vi "auto auger.vi"(3 "Number of Frisbees":i8, 4 "Index Down":bool, 5 "Index Up":bool) -> (0 "Number of Frisbees Out":i8, 1 "Setpoint Out":dbl format="%.2f", 2 "Finished":bool)   [LabVIEW 2012]
uses:
  typedefs/subStates.ctl
  <vilib>/addons/control/pid/NI_PID_pid.lvlib
  <vilib>/addons/control/pid/pid.llb/PID (DBL).vi
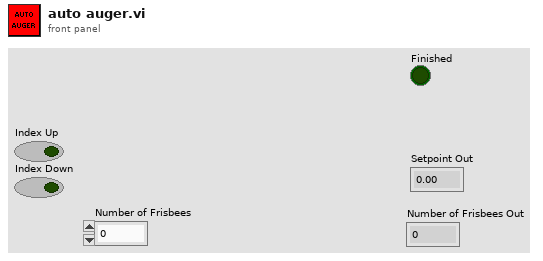
[diagram p1: front panel]
types:
  T1 = typedef "subStates.ctl" = enum16{"null", "wait", "driver control", "auto", "manual override", "hold position", "rotate", "feeder", "shoot", "end"}
  T2 = typedef "WPI_DigitalInputDevRef.ctl" = cluster{"DevStatus":errorcluster, "DIO Channel":T3, "Digital Module":T4}
  T3 = typedef "FPGA_DIOChannel.ctl" = enum8{"DIO 1", "DIO 2", "DIO 3", "DIO 4", "DIO 5", "DIO 6", "DIO 7", "DIO 8", "DIO 9", "DIO 10", "DIO 11", "DIO 12", "DIO 13", "DIO 14", "Invalid"}
  T4 = typedef "FPGA_TypedefDigitalModule.ctl" = enum16{"Digital Module 1", "Digital Module 2"}
  T5 = typedef "WPI_EncoderDevRef.ctl" = cluster{"DevStatus":errorcluster, "EncoderIndex":T6, "CounterIndex":T7, "DistancePerCount":dbl, "Decoding Type":T8}
  T6 = typedef "FPGA_EncoderIdx.ctl" = enum8{"Enc 0", "Enc 1", "Enc 2", "Enc 3", "Invalid"}
  T7 = typedef "FPGA_CounterCtrSystemIndex.ctl" = enum8{"Ctr 0", "Ctr 1", "Ctr 2", "Ctr 3", "Ctr 4", "Ctr 5", "Ctr 6", "Ctr 7", "Invalid"}
  T8 = typedef "WPI_EncoderType.ctl" = enum16{"1x", "2x", "4x"}
  T9 = cluster{"proportional gain (Kc)":dbl, "integral time (Ti, min)":dbl, "derivative time (Td, min)":dbl}
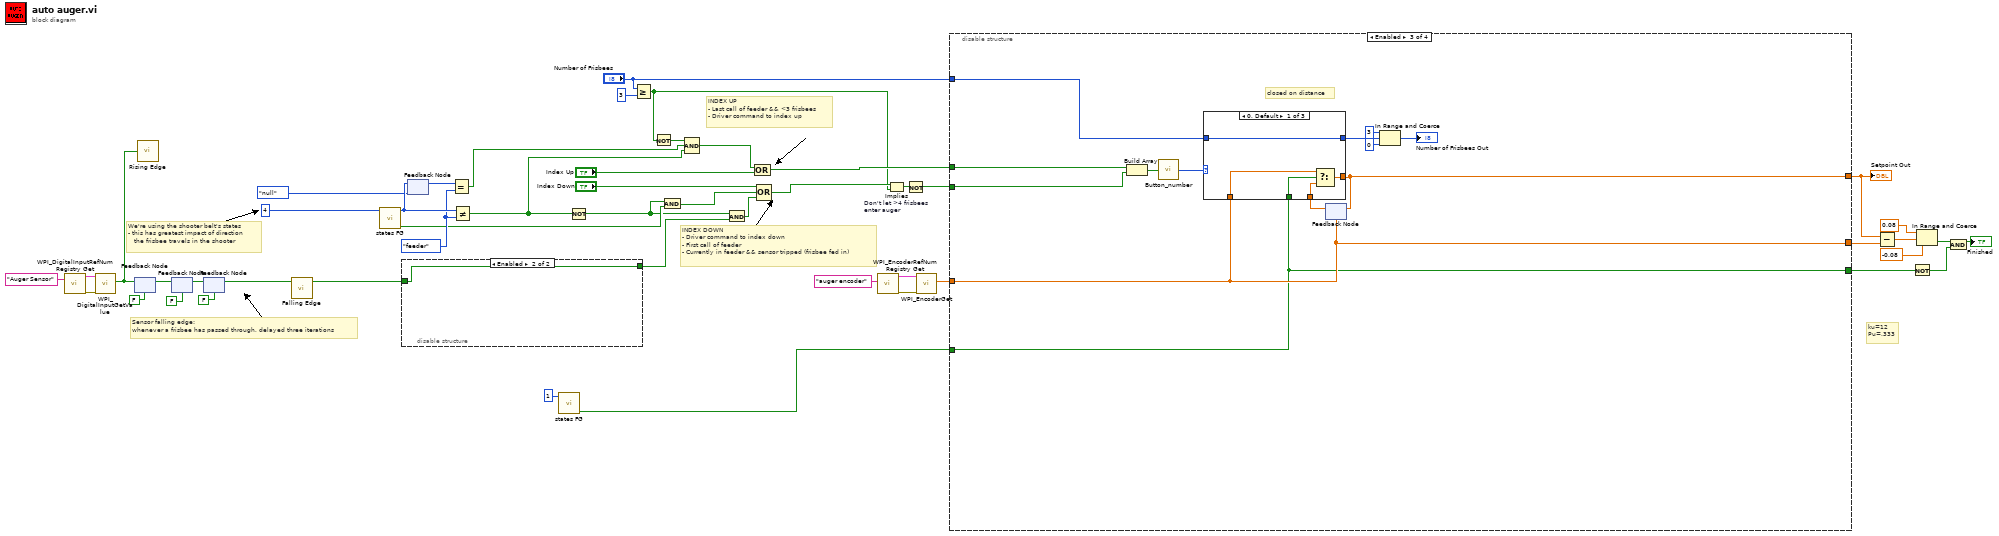
[diagram p0: block diagram]
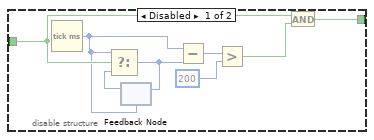
[diagram p2: hidden frame]
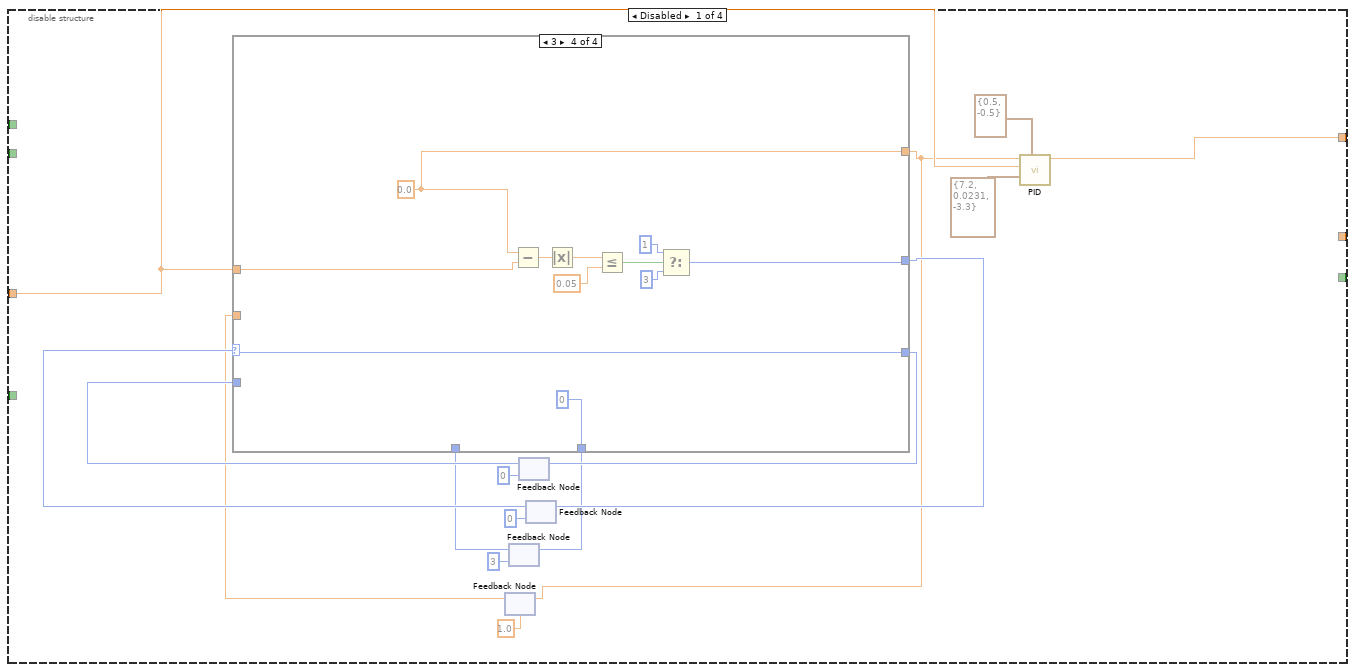
[diagram p3: hidden frame]
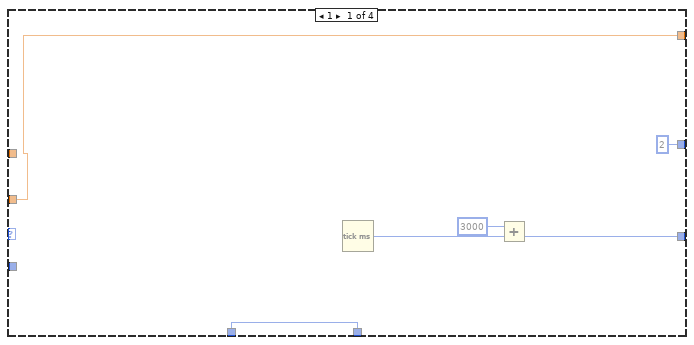
[diagram p4: hidden frame]
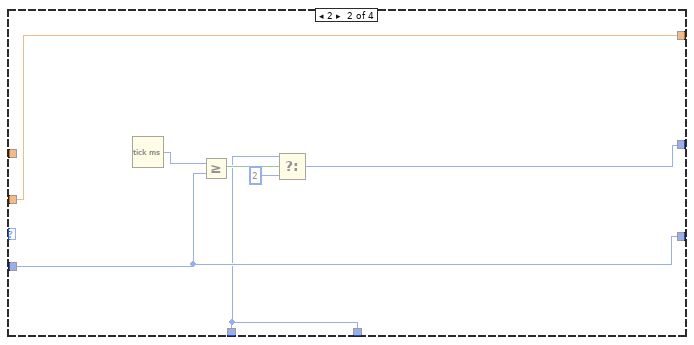
[diagram p5: hidden frame]
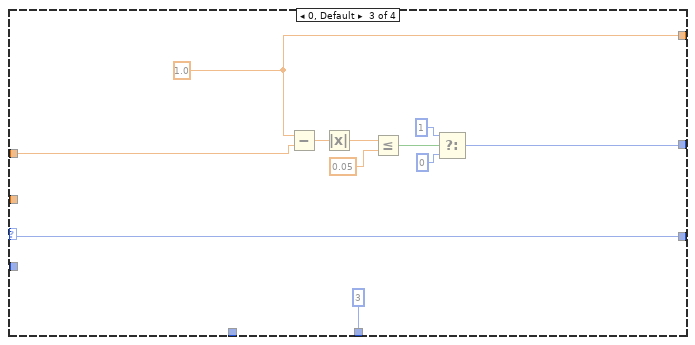
[diagram p6: hidden frame]
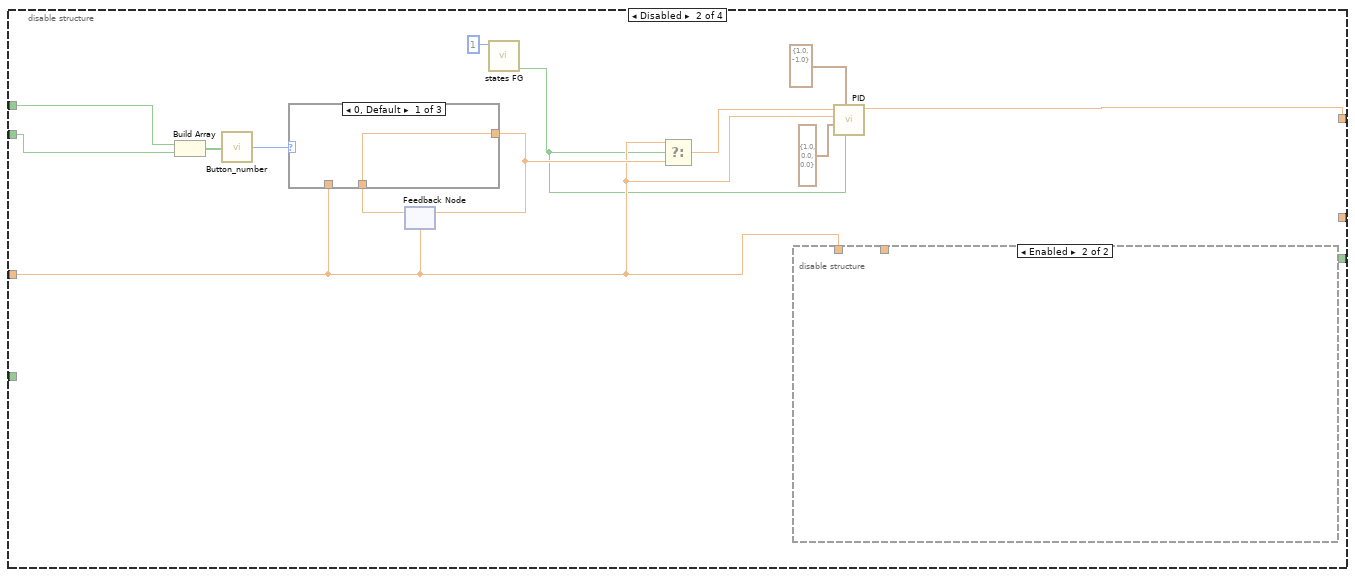
[diagram p7: hidden frame]
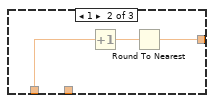
[diagram p8: hidden frame]
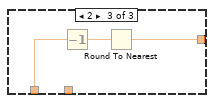
[diagram p9: hidden frame]
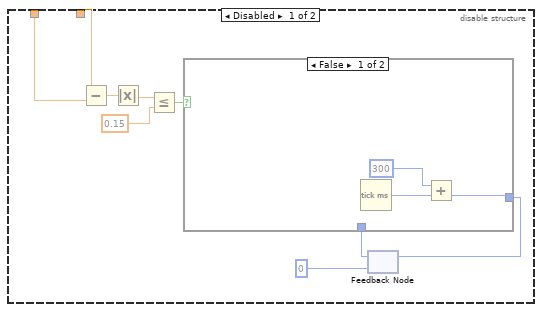
[diagram p10: hidden frame]
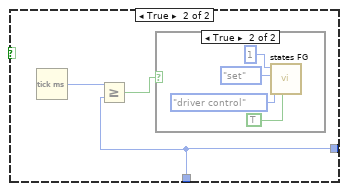
[diagram p11: hidden frame]
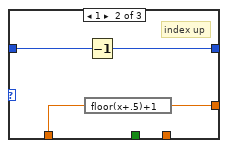
[diagram p13: hidden frame]
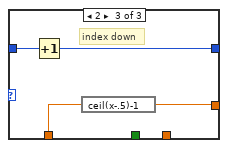
[diagram p14: hidden frame]
diagram:
  w36 = subStates."feeder" ("x")
  # "Sensor falling edge:\nwhenever a frisbee has passed through, delayed three iterations"
  # "We're using the shooter belt's states\n- this has greatest impact of direction\n   the frisbee travels in the shooter"
  # "INDEX DOWN\n- Driver command to index down\n- First call of feeder\n- Currently in feeder && sensor tripped (frisbee fed in)"
  # "INDEX UP\n- Last call of feeder && <3 frisbees\n- Driver command to index up"
  # "ku=12\nPu=.333"
  n1 = call <vilib>:"WPI_DigitalInputRefNum Registry Get.vi"("refnum name"="Auger Sensor") -> ("error out"=w42:errorcluster, "DigitalInputDevRef"=w41:T2)  [unwired: 9 in]
  n2 = call <vilib>:"WPI_DigitalInputGetValue.vi"("error in (no error)"=w42, "DigitalInputDevRef"=w41) -> ("Value"=w15:bool)  [unwired: 7 in, 2 out]
  n3 = feedback-in #1(w15) -> ()
  n4 = feedback #1(FALSE) -> (w19:bool)
  n5 = call "Rising Edge.vi"("Input"=w15) -> ()  [unwired: 1 out]
  n6 = feedback #2(FALSE) -> (w17:bool)
  n7 = feedback-in #2(w19) -> ()
  n8 = feedback #3(FALSE) -> (w16:bool)
  n9 = feedback-in #3(w17) -> ()
  n10 = call "Falling Edge.vi"("Input"=w16) -> ("Output"=w22:bool)  [unwired: 4 in]
  n11 = call "states FG.vi"("Loop ID"=4) -> ("first call?"=w32:bool, "subState out"=w39:T1)  [unwired: 7 in, 2 out]
  n12 = disable-structure shown="Enabled" {
    disable-tunnel: w22 -> [w56 w58]
    disable-tunnel: [w50 w58] -> w21
    frame Disabled {
      n13 = Tick Count (ms)() -> (millisecond timer value=w54:u32)
      n14 = feedback #4(w54) -> (w57:u32)
      n15 = Select(t=w54, s=w56, f=w57) -> (s? t:f=w55:u32)
      n16 = feedback-in #4(w55) -> ()
      n17 = Subtract(x=w54, y=w55) -> (x-y=w53:u32)
      n18 = Greater?(x=w53, y=u32 200) -> (0:w51:bool)
      n19 = And(x=w56, y=w51) -> (x .and. y?=w50:bool)
    }
    frame Enabled {
    }
  }
  n20 = feedback-in #5(w39) -> ()
  n21 = feedback #5(subStates."null" ("x")) -> (w37:T1)
  n22 = Equal?(x=w37, y=w36) -> (x = y?=w28:bool)
  n23 = Not Equal?(x=w39, y=w36) -> (x != y?=w29:bool)
  n24 = call "states FG.vi"("Loop ID"=1) -> ("first call?"=w3:bool)  [unwired: 7 in, 3 out]
  n25 = Not(x=w29) -> (.not. x?=w31:bool)
  n26 = Greater Or Equal?(x="Number of Frisbees", y=i8 3) -> (x >= y?=w26:bool)
  n27 = Not(x=w26) -> (.not. x?=w27:bool)
  n28 = And(x=w31, y=w32) -> (x .and. y?=w30:bool)
  n29 = Compound Arithmetic op=AND(w27, w28, w29) -> (w23:bool)
  n30 = And(x=w31, y=w21) -> (x .and. y?=w33:bool)
  n31 = Compound Arithmetic op=OR(w23, "Index Up") -> (w40:bool)
  n32 = Compound Arithmetic op=OR("Index Down", w30, w33) -> (w44:bool)
  n33 = call <vilib>:"WPI_EncoderRefNum Registry Get.vi"("refnum name"="auger encoder") -> ("error out"=w47:errorcluster, "EncoderDevRef"=w48:T5)  [unwired: 9 in]
  n34 = Implies "Don't let >4 frisbees enter auger"(1:w26, 2:w44) -> (0:w35:bool)
  n35 = Not(x=w35) -> (.not. x?=w25:bool)
  n36 = call <vilib>:"WPI_EncoderGet.vi"("error in (no error)"=w47, "EncoderDevRef"=w48) -> ("Distance"=w46:dbl)  [unwired: 4 in, 5 out]
  n37 = disable-structure shown="Enabled" {
    disable-tunnel: [w63 w113 w151 _] -> w13
    disable-tunnel: w46 -> [w62 w116 w150 _]
    disable-tunnel: w40 -> [_ w111 w158 _]
    disable-tunnel: w25 -> [_ w110 w157 _]
    disable-tunnel: "Number of Frisbees" -> [_ _ w155 _]
    disable-tunnel: [_ _ w150 _] -> w12
    disable-tunnel: [_ _ w149 _] -> w6
    disable-tunnel: w3 -> [_ _ w149 _]
    frame Disabled {
      n38 = feedback #6(1.0) -> (w60:dbl)
      n39 = feedback #7(3) -> (w68:i32)
      n40 = feedback #8(u32 0 ("millisecond timer value")) -> (w71:u32)
      n41 = feedback #9(u32 0 ("millisecond timer value")) -> (w74:u32)
      n42 = case shown="3" w74 {
        tunnel: [u32 2 ("millisecond timer value") w84 w96 w104] -> w73
        tunnel: [w79 w85 w95 w103] -> w72
        tunnel: w71 -> [_ w85 w95 w103]
        tunnel: w68 -> [w76 w83 _ _]
        tunnel: [w76 w83 3 0] -> w67
        tunnel: w62 -> [_ _ w89 w99]
        tunnel: [w75 w81 w88 w100] -> w59
        tunnel: w60 -> [w75 w81 _ _]
        frame 1 {
          n43 = Tick Count (ms)() -> (millisecond timer value=w80:u32)
          n44 = Add(x=u32 3000, y=w80) -> (x+y=w79:u32)
        }
        frame 2 {
          n45 = Tick Count (ms)() -> (millisecond timer value=w87:u32)
          n46 = Greater Or Equal?(x=w87, y=w85) -> (x >= y?=w86:bool)
          n47 = Select(t=w83, s=w86, f=2) -> (s? t:f=w84:i32)
        }
        frame 0, Default {
          w88 = 1.0 ("setpoint")
          n48 = Subtract(x=w88, y=w89) -> (x-y=w92:dbl)
          n49 = Absolute Value(x=w92) -> (abs(x)=w90:dbl)
          n50 = Less Or Equal?(x=w90, y=0.05) -> (x <= y?=w97:bool)
          n51 = Select(t=u32 1 ("millisecond timer value"), s=w97, f=u32 0 ("millisecond timer value")) -> (s? t:f=w96:u32)
        }
        frame 3 {
          w100 = 0.0 ("setpoint")
          n52 = Subtract(x=w100, y=w99) -> (x-y=w105:dbl)
          n53 = Absolute Value(x=w105) -> (abs(x)=w101:dbl)
          n54 = Less Or Equal?(x=w101, y=0.05) -> (x <= y?=w108:bool)
          n55 = Select(t=u32 1 ("millisecond timer value"), s=w108, f=u32 3 ("millisecond timer value")) -> (s? t:f=w104:u32)
        }
      }
      n56 = feedback-in #6(w59) -> ()
      n57 = feedback-in #7(w67) -> ()
      n58 = feedback-in #8(w72) -> ()
      n59 = feedback-in #9(w73) -> ()
      n60 = call-poly <vilib>:"PID.vi"("output range"=cluster{"output high":dbl, "output low":dbl} {"output high"=0.5, "output low"=-0.5}, "PID gains"=T9 {"proportional gain (Kc)"=7.2, "integral time (Ti, min)"=0.0231, "derivative time (Td, min)"=-3.3}, "process variable"=w62, "setpoint"=w59) -> ("output"=w63:dbl)  [unwired: 6 in, 1 out]
    }
    frame Disabled {
      n61 = Build Array(w111, w110) -> (w121:bool[])
      n62 = call "Button_number.vi"("Button Array"=w121) -> ("Button Pressed"=w120:i32)
      n63 = feedback #10(w116) -> (w118:dbl)
      n64 = case shown="0, Default" w120 {
        tunnel: w116 -> [_ w126 w129]
        tunnel: [w123 w124 w127] -> w119
        tunnel: w118 -> [w123 _ _]
        frame 0, Default {
        }
        frame 1 {
          n65 = Increment(x=w126) -> (x+1=w125:dbl)
          n66 = Round To Nearest(number=w125) -> (nearest integer value=w124:dbl)
        }
        frame 2 {
          n67 = Decrement(x=w129) -> (x-1=w128:dbl)
          n68 = Round To Nearest(number=w128) -> (nearest integer value=w127:dbl)
        }
      }
      n69 = feedback-in #10(w119) -> ()
      n70 = call "states FG.vi"("Loop ID"=1) -> ("first call?"=w112:bool)  [unwired: 7 in, 3 out]
      n71 = Select(t=w116, s=w112, f=w119) -> (s? t:f=w117:dbl)
      n72 = disable-structure shown="Enabled" {
        disable-tunnel: w116 -> [w137 _]
        disable-tunnel: _ -> [w130 _]
        frame Disabled {
          n73 = Subtract(x=w130, y=w137) -> (x-y=w138:dbl)
          n74 = Absolute Value(x=w138) -> (abs(x)=w136:dbl)
          n75 = Less Or Equal?(x=w136, y=0.15) -> (x <= y?=w134:bool)
          n76 = feedback #11(u32 0 ("millisecond timer value")) -> (w131:u32)
          n77 = case shown="False" w134 {
            tunnel: [w140 w143] -> w133
            tunnel: w131 -> [_ w143]
            frame False {
              n78 = Tick Count (ms)() -> (millisecond timer value=w141:u32)
              n79 = Add(x=u32 300 ("settling time (ms)"), y=w141) -> (x+y=w140:u32)
            }
            frame True {
              n80 = Tick Count (ms)() -> (millisecond timer value=w144:u32)
              n81 = Greater Or Equal?(x=w144, y=w143) -> (x >= y?=w142:bool)
              n82 = case shown="True" w142 {
                frame False {
                }
                frame True {
                  n83 = call "states FG.vi"("exit in"=TRUE, "subState in"=subStates."driver control", "menu (get)"=enum16{"set", "get"}."set", "Loop ID"=1) -> ()  [unwired: 4 in, 4 out]
                }
              }
            }
          }
          n84 = feedback-in #11(w133) -> ()
        }
        frame Enabled {
        }
      }
      n85 = call-poly <vilib>:"PID.vi"("reinitialize? (F)"=w112, "output range"=cluster{"output high":dbl, "output low":dbl} {"output high"=1.0, "output low"=-1.0}, "PID gains"=T9 {"proportional gain (Kc)"=1.0, "integral time (Ti, min)"=0.0, "derivative time (Td, min)"=0.0}, "process variable"=w116, "setpoint"=w117) -> ("output"=w113:dbl)  [unwired: 5 in, 1 out]
    }
    frame Enabled {
      # "closed on distance"
      n86 = Build Array(w158, w157) -> (w160:bool[])
      n87 = call "Button_number.vi"("Button Array"=w160) -> ("Button Pressed"=w159:i32)
      n88 = feedback #12(w150) -> (w161:dbl)
      n89 = case shown="0, Default" w159 {
        tunnel: w150 -> [w163 w168 w172]
        tunnel: [w165 w167 w171] -> w151
        tunnel: w161 -> [w164 _ _]
        tunnel: [w166 w169 w173] -> w156
        tunnel: w155 -> [w166 w170 w174]
        tunnel: w149 -> [w162 _ _]
        frame 0, Default {
          n90 = Select(t=w163, s=w162, f=w164) -> (s? t:f=w165:dbl)
        }
        frame 1 {
          # "index up"
          n91 = expression code="floor(x+.5)+1"(w168) -> (w167:dbl)
          n92 = Decrement(x=w170) -> (x-1=w169:i8)
        }
        frame 2 {
          # "index down"
          n93 = Increment(x=w174) -> (x+1=w173:i8)
          n94 = expression code="ceil(x-.5)-1"(w172) -> (w171:dbl)
        }
      }
      n95 = feedback-in #12(w151) -> ()
      n96 = In Range and Coerce(upper limit=i8 3, x=w156, lower limit=i8 0 ("x")) -> (coerced(x)=→"Number of Frisbees Out":i8)  [unwired: 1 out]
    }
    frame Disabled {
    }
  }
  "Setpoint Out" <- w13
  n97 = Subtract(x=w13, y=w12) -> (x-y=w11:dbl)
  n98 = Not(x=w6) -> (.not. x?=w5:bool)
  n99 = In Range and Coerce(upper limit=0.08, x=w11, lower limit=-0.08) -> (In Range?=w8:bool)  [unwired: 1 out]
  n100 = And(x=w8, y=w5) -> (x .and. y?=→"Finished":bool)
